vi "Get Magnet Field.vi"(4 "Axis":T1, 8 "error in (no error)":errorcluster, 11 "IPS120 in":refnum<class "IPS120.lvclass">) -> (0 "error out":errorcluster, 1 "Status":variant, 2 "B Field (T)":dbl, 3 "IPS120 out":refnum<class "IPS120.lvclass">)   [LabVIEW 2016, in "IPS120.lvclass"]
uses:
  IPS120.lvclass
  <userlib>/LevyLab/Levylab Instruments/Instrument Types/Cryostat/Typedefs/Magnet Axis--Enum.ctl
  API/IPS-120-API.lvlib
  <userlib>/LevyLab/Levylab Instruments/Instrument Types/Cryostat/Instrument.Cryostat.lvclass
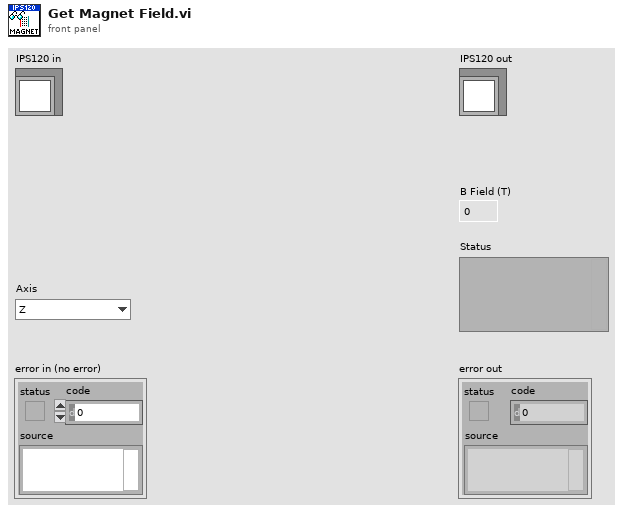
[diagram p1: front panel]
types:
  T1 = typedef "Instrument.Cryostat.lvclass/Magnet Axis--Enum.ctl" = enum16{"Z", "X", "Y"}
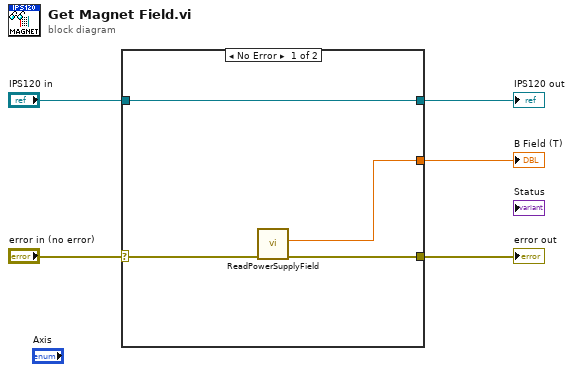
[diagram p0: block diagram]
diagram:
  n1 = case shown="No Error" "error in (no error)" {
    selector: "error in (no error)" -> [w8 w10]
    tunnel: [w7 w10] -> w5
    tunnel: [w9 _] -> w4
    tunnel: [w6 w11] -> w3
    tunnel: "IPS120 in" -> [w6 w11]
    frame No Error {
      n2 = call "ReadPowerSupplyField.vi"("error in"=w8) -> ("error out"=w7:errorcluster, "Power Supply Field (T)"=w9:dbl)  [unwired: 9 in]
    }
    frame Error {
    }
  }
  "error out" <- w5
  "IPS120 out" <- w3
  "B Field (T)" <- w4
